vi "close.vi"(8 "error in":errorcluster, 11 "module in":refnum<class "AppStateMachine runtime.lvclass">) -> (0 "error out":errorcluster)   [LabVIEW 2017, in "AppStateMachine runtime.lvclass"]
doc: "Provides an interface for terminating a module instance. While this interface performs no operations, a child should close and deallocate any open references or memory."
uses:
  AppStateMachine runtime.lvclass
  AppStateMachine runtime.lvclass/AppStateMachine runtime.ctl
  <vilib>/NI/NI JSONRPC Server Framework/Classes/Server/JSONRPC Server.lvclass
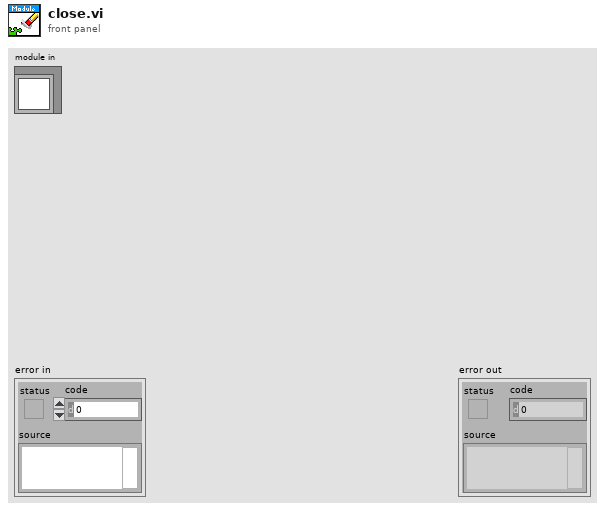
[diagram p1: front panel]
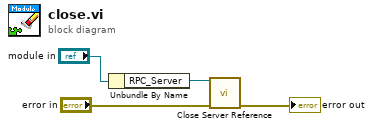
[diagram p0: block diagram]
diagram:
  n1 = Unbundle By Name("module in") -> ("RPC_Server"=w2:refnum<class "JSONRPC Server.lvclass">)
  n2 = call-dynamic "Close Server Reference.vi"("error in (no error)"="error in", "Server in"=w2) -> ("error out"=→"error out":errorcluster)  [unwired: 9 in]
